vi "Trim Array Whitespace.vi"(11 "Array in":string[](array[string])) -> (3 "Array out":string[](array[string]))   [LabVIEW 2021]
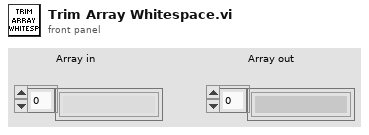
[diagram p1: front panel]
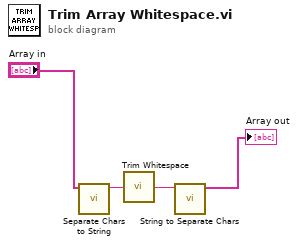
[diagram p0: block diagram]
diagram:
  n1 = call "Separate Chars to String.vi"("Array"="Array in") -> ("String"=w2:string)  [unwired: 10 in]
  n2 = call <vilib>:"Trim Whitespace.vi"("string"=w2) -> ("trimmed string"=w3:string)  [unwired: 1 in]
  n3 = call "String to Separate Chars.vi"("String"=w3) -> ("Array"=→"Array out":string[])  [unwired: 10 in]
